vi "Router - Writer.vi"(8 "error in (no error)":errorcluster, 11 "Router Data In":T1) -> (0 "error out":errorcluster, 3 "Router Data Out":T1)   [LabVIEW 2016, in "PXImc Router.lvlib"]
uses:
  PXImc Router.lvlib
  Controls/Router - Configuration.ctl
  Controls/Target Type.ctl
  Controls/Router/Node Block R-W Properties.ctl
  Controls/Router/Block Properties.ctl
  Controls/Router/Router - PXImc Properties.ctl
  Controls/Router/Router - PXImc Card Properties.ctl
  <vilib>/pximc/nipximc.lvlib
  <vilib>/pximc/Acquire Write Region (DBL).vi
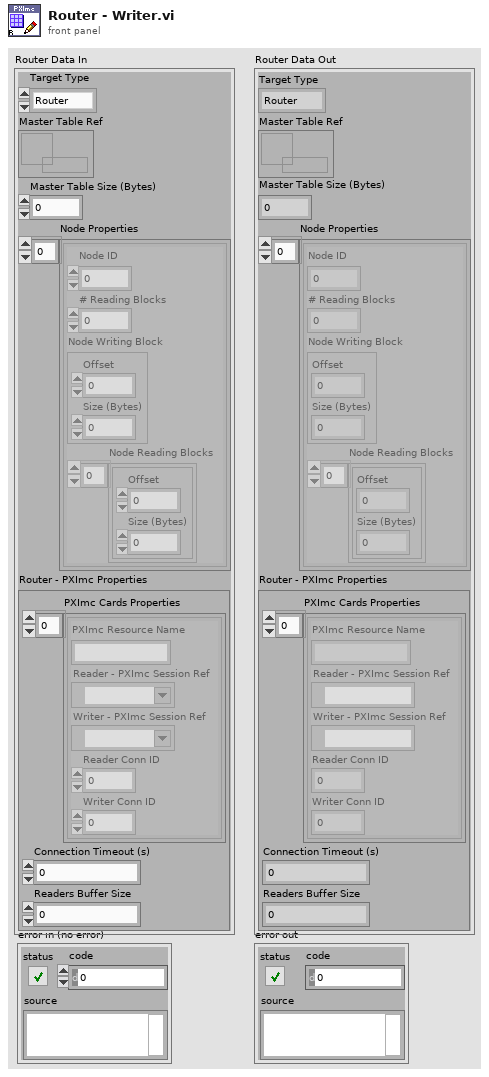
[diagram p1: front panel]
types:
  T1 = typedef "PXImc Router.lvlib/Router - Configuration.ctl" = cluster{"Target Type":T2, "Master Table Ref":refnum<data-value>, "Master Table Size (Bytes)":u32, "Node Properties":T3[], "Router - PXImc Properties":T5}
  T2 = typedef "PXImc Router.lvlib/Target Type.ctl" = enum16{"Router", "Node"}
  T3 = typedef "PXImc Router.lvlib/Node Block R-W Properties.ctl" = cluster{"Node ID":u32, "# Reading Blocks":u32, "Node Writing Block":T4, "Node Reading Blocks":T4[]}
  T4 = typedef "PXImc Router.lvlib/Block Properties.ctl" = cluster{"Offset":u32, "Size (Bytes)":u32}
  T5 = typedef "PXImc Router.lvlib/Router - PXImc Properties.ctl" = cluster{"PXImc Cards Properties":T6[], "Connection Timeout (s)":dbl, "Readers Buffer Size":u64}
  T6 = typedef "PXImc Router.lvlib/Router - PXImc Card Properties.ctl" = cluster{"PXImc Resource Name":string, "Reader - PXImc Session Ref":refnum<k21>, "Writer - PXImc Session Ref":refnum<k21>, "Reader Conn ID":u16, "Writer Conn ID":u16}
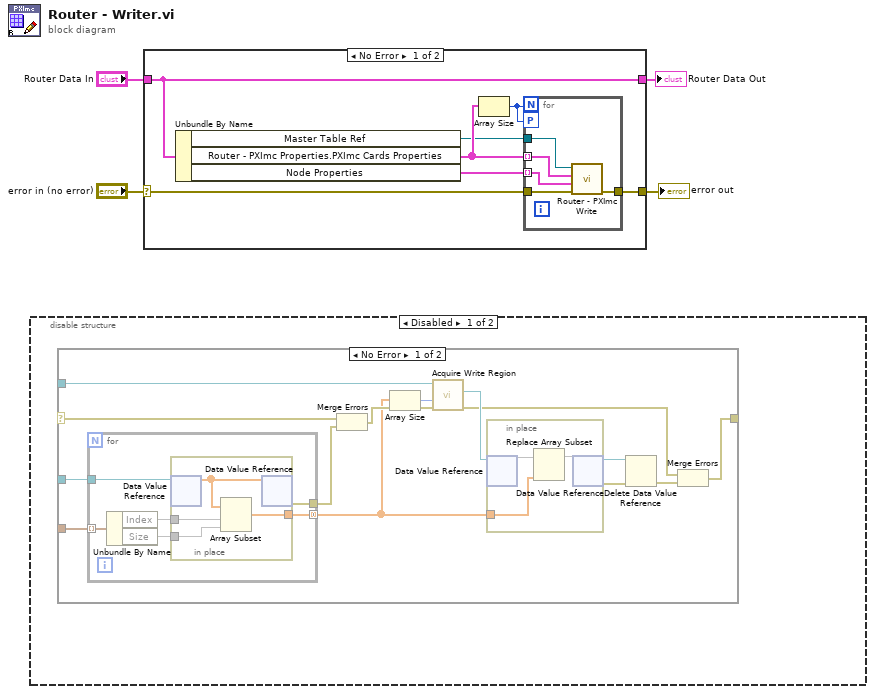
[diagram p0: block diagram]
diagram:
  n1 = disable-structure shown="Disabled" {
    frame Disabled {
      n2 = case shown="No Error" {
        selector: _ -> [w15 w32]
        tunnel: _ -> [w18 _]
        tunnel: _ -> [w17 _]
        tunnel: [w16 w32] -> _
        tunnel: _ -> [w14 _]
        frame No Error {
          n3 = for {
            tunnel: w17 -> [w24]
            tunnel: w14 -> [w23] mode=indexing
            tunnel: [w22] -> w7
            tunnel: [w19] -> w5 mode=concatenating
            n4 = Unbundle By Name(w23) -> ("Index"=w21, "Size"=w20)
            n5 = in-place {
              in-place-border: [w27] -> w19
              in-place-border: w21 -> [w26]
              in-place-border: w20 -> [w28]
              n6 = in-place-dvr #1(w24) -> (w25:dbl[])  [unwired: 1 out]
              n7 = Array Subset(array=w25, index=w26, length=w28) -> (w27:dbl[])
              n8 = in-place-dvr #1(w25) -> (w22:errorcluster)  [unwired: 1 out]
            }
          }
          n9 = Merge Errors(w15, w7) -> (w6:errorcluster)
          n10 = Array Size(array=w5) -> (size(s)=w8:i32)
          n11 = call-poly <vilib>:"Acquire Write Region.vi"("error in (no error)"=w6, "number of elements"=w8, "session in"=w18) -> ("error out"=w9:errorcluster, "write region reference"=w10:refnum<data-value>)  [unwired: 5 in, 2 out]
          n12 = in-place {
            in-place-border: w5 -> [w29]
            n13 = in-place-dvr #2(w10) -> (w31:dbl[])  [unwired: 1 out]
            n14 = Replace Array Subset(array=w31, new element=w29) -> (w30:dbl[])  [unwired: 1 in]
            n15 = in-place-dvr #2(w30) -> (w11:refnum<data-value>, w13:errorcluster)
          }
          n16 = Delete Data Value Reference(data value reference=w11, error in=w13) -> (error out=w12:errorcluster)  [unwired: 1 out]
          n17 = Merge Errors(w9, w12) -> (w16:errorcluster)
        }
        frame Error {
        }
      }
    }
    frame Enabled {
    }
  }
  n18 = case shown="No Error" "error in (no error)" {
    selector: "error in (no error)" -> [w39 w46]
    tunnel: [w33 w46] -> w3
    tunnel: "Router Data In" -> [w38 w45]
    tunnel: [w38 w45] -> w1
    frame No Error {
      n19 = Unbundle By Name(w38) -> ("Master Table Ref"=w34:refnum<data-value>, "Router - PXImc Properties.PXImc Cards Properties"=w36:T6[], "Node Properties"=w37:T3[])
      n20 = Array Size(array=w36) -> (size(s)=w35:i32)
      n21 = for {
        N: w35 -> [_]
        tunnel: w37 -> [w40] mode=indexing
        tunnel: w36 -> [w41] mode=indexing
        workers-P: w35 -> [_]
        tunnel: w39 -> [w43]
        tunnel: w34 -> [w44]
        tunnel: [w42] -> w33
        n22 = call "Router - PXImc Write.vi"("error in (no error)"=w43, "Node Properties"=w40, "PXImc Cards Properties"=w41, "Master Table Ref"=w44) -> ("error out"=w42:errorcluster)  [unwired: 7 in]
      }
    }
    frame Error {
    }
  }
  "error out" <- w3
  "Router Data Out" <- w1
